vi "Get All Child Node Addresses by Address.vi"(8 "error in":errorcluster, 10 "Address":i32[](array[numeric]), 11 "XML Document in":refnum<class "XML Document.lvclass">) -> (0 "error out":errorcluster, 1 "String Addresses":string[](array[string]), 2 "Addresses":i32[][](array[numeric]), 3 "XML Document out":refnum<class "XML Document.lvclass">)   [LabVIEW 2014, in "XML Document.lvclass"]
uses:
  XML Document.lvclass
  Node_class/Node.lvclass
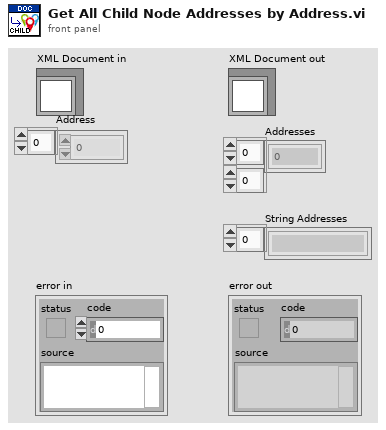
[diagram p1: front panel]
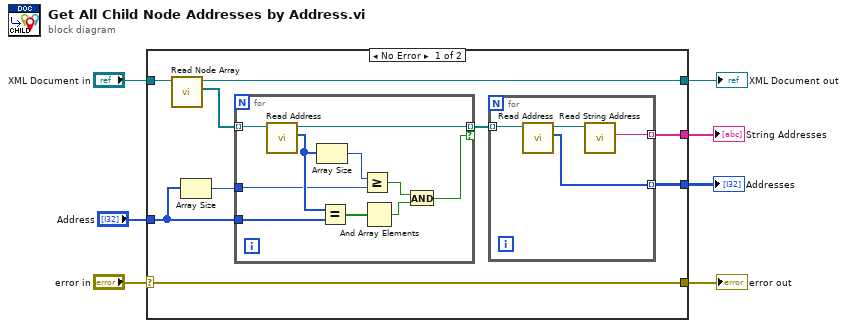
[diagram p0: block diagram]
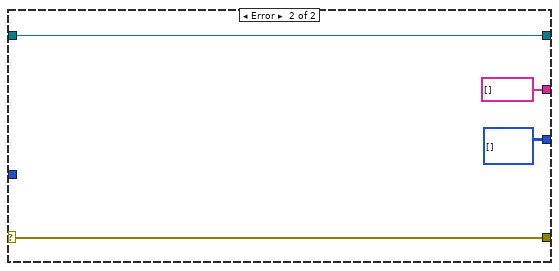
[diagram p2: hidden frame]
diagram:
  n1 = case shown="No Error" "error in" {
    selector: "error in" -> [w15 w34]
    tunnel: [w15 w34] -> w6
    tunnel: [w14 w33] -> w4
    tunnel: "XML Document in" -> [w16 w33]
    tunnel: "Address" -> [w12 _]
    tunnel: [w9 string[] []] -> w2
    tunnel: [w8 i32[][] [] ("Address")] -> w1
    frame No Error {
      n2 = call-dynamic "Read Node Array.vi"("XML Document in"=w16) -> ("Node Array"=w13:refnum<class "Node.lvclass">[], "XML Document out"=w14:refnum<class "XML Document.lvclass">)  [unwired: 8 in, 1 out]
      n3 = Array Size(array=w12) -> (size(s)=w11:i32)
      n4 = for {
        tunnel: w13 -> [w30] mode=indexing
        tunnel: w12 -> [w29]
        tunnel: w11 -> [w26]
        tunnel: [w22] -> w10 mode=indexing if=w21
        n5 = call-dynamic "Read Address.vi"("Node in"=w30) -> ("Address"=w28:i32[], "Node out"=w22:refnum<class "Node.lvclass">)  [unwired: 8 in, 1 out]
        n6 = Array Size(array=w28) -> (size(s)=w27:i32)
        n7 = Equal?(x=w28, y=w29) -> (x = y?=w25:bool[])
        n8 = Greater Or Equal?(x=w27, y=w26) -> (x >= y?=w23:bool)
        n9 = And Array Elements(Boolean array=w25) -> (logical AND=w24:bool)
        n10 = And(x=w23, y=w24) -> (x .and. y?=w21:bool)
      }
      n11 = for {
        tunnel: w10 -> [w20] mode=indexing
        tunnel: [w18] -> w8 mode=indexing
        tunnel: [w17] -> w9 mode=indexing
        n12 = call-dynamic "Read Address.vi"("Node in"=w20) -> ("Address"=w18:i32[], "Node out"=w19:refnum<class "Node.lvclass">)  [unwired: 8 in, 1 out]
        n13 = call-dynamic "Read String Address.vi"("Node in"=w19) -> ("String Address"=w17:string)  [unwired: 8 in, 2 out]
      }
    }
    frame Error {
    }
  }
  "error out" <- w6
  "XML Document out" <- w4
  "String Addresses" <- w2
  "Addresses" <- w1
